vi "Test Data.vi"(1 "Size":i32=1) -> (0 "Data":variant)   [LabVIEW 2019, in "LV-Data.PGSQL.lvclass"]
uses:
  LV-Data.PGSQL.lvclass
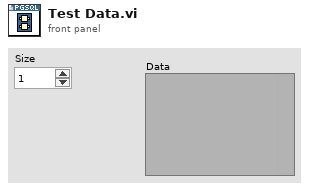
[diagram p1: front panel]
types:
  T1 = cluster{"integer label":i32, "float label":dbl, "string label":string, "boolean label":bool, "timestamp label":timestamp}
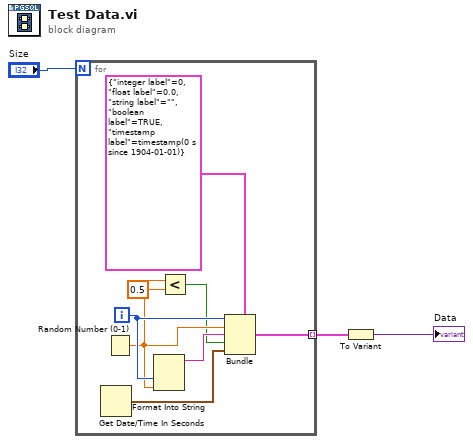
[diagram p0: block diagram]
diagram:
  n1 = for {
    N: "Size" -> [_]
    tunnel: [w4] -> w2 mode=indexing
    i -> [w11]
    n2 = Get Date/Time In Seconds() -> (seconds since 1Jan1904=w10:timestamp)
    n3 = Random Number (0-1)() -> (number: 0 to 1=w8:dbl)
    n4 = Format Into String(w11, w8) -> (resulting string=w9:string)  [unwired: 3 in, 1 out]
    n5 = Less?(x=w8, y=0.5) -> (x < y?=w6:bool)
    n6 = Bundle(cluster=T1 {"integer label"=0, "float label"=0.0, "string label"="", "boolean label"=TRUE, "timestamp label"=timestamp(0 s since 1904-01-01)}, "integer label"=w11, "float label"=w8, "string label"=w9, "boolean label"=w6, "timestamp label"=w10) -> (w4:T1)
  }
  n7 = To Variant(anything=w2) -> (Variant=→"Data":variant)
